vi "RT main.vi"() -> ()   [LabVIEW 2018]
uses:
  <vilib>/userdefined/High Color/nirio_resource_hc.ctl
  controls/Controller Data.ctl
  RT-FPGA Interface API/RT-FPGA Interface API.lvlib
panel:
  out "# pending remove":i32
  out "# elements in queue":i32
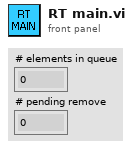
[diagram p1: front panel]
types:
  T1 = typedef "Controller Data.ctl" = cluster{"Closed Loop Enabled":bool, "Proportional valve 1":dbl, "Proportional valve 2":dbl, "Plant Control Variables":cluster{"Tank 1 Level":dbl, "Tank 2 Level":dbl, "Tank 3 Level":dbl, "Tank 4 Level":dbl, "Pump 1":dbl, "Pump 2":dbl}, "Setpoints":cluster{"Setpoint tank 1":dbl, "Setpoint tank 2":dbl}, "Controller":cluster{"A":dbl[][], "B":dbl[][], "C":dbl[][], "D":dbl[][]}}
  T2 = typedef "nirio_resource_hc.ctl" = tag
  T3 = typedef "RT-FPGA Interface API.lvlib/FPGA ref.ctl" = refnum<k20>
  T4 = cluster{"Proportional valve 1":dbl, "Proportional valve 2":dbl, "Pump 1":dbl, "Pump 2":dbl}
  T5 = cluster{"Setpoint Tank 1":dbl, "Setpoint Tank 2":dbl}
  T6 = cluster{"A":dbl[][], "B":dbl[][], "C":dbl[][], "D":dbl[][]}
  T7 = cluster{"Setpoint tank 1":dbl, "Setpoint tank 2":dbl}
  T8 = cluster{"Tank 1 Level":dbl, "Tank 2 Level":dbl, "Tank 3 Level":dbl, "Tank 4 Level":dbl, "Pump 1":dbl, "Pump 2":dbl}
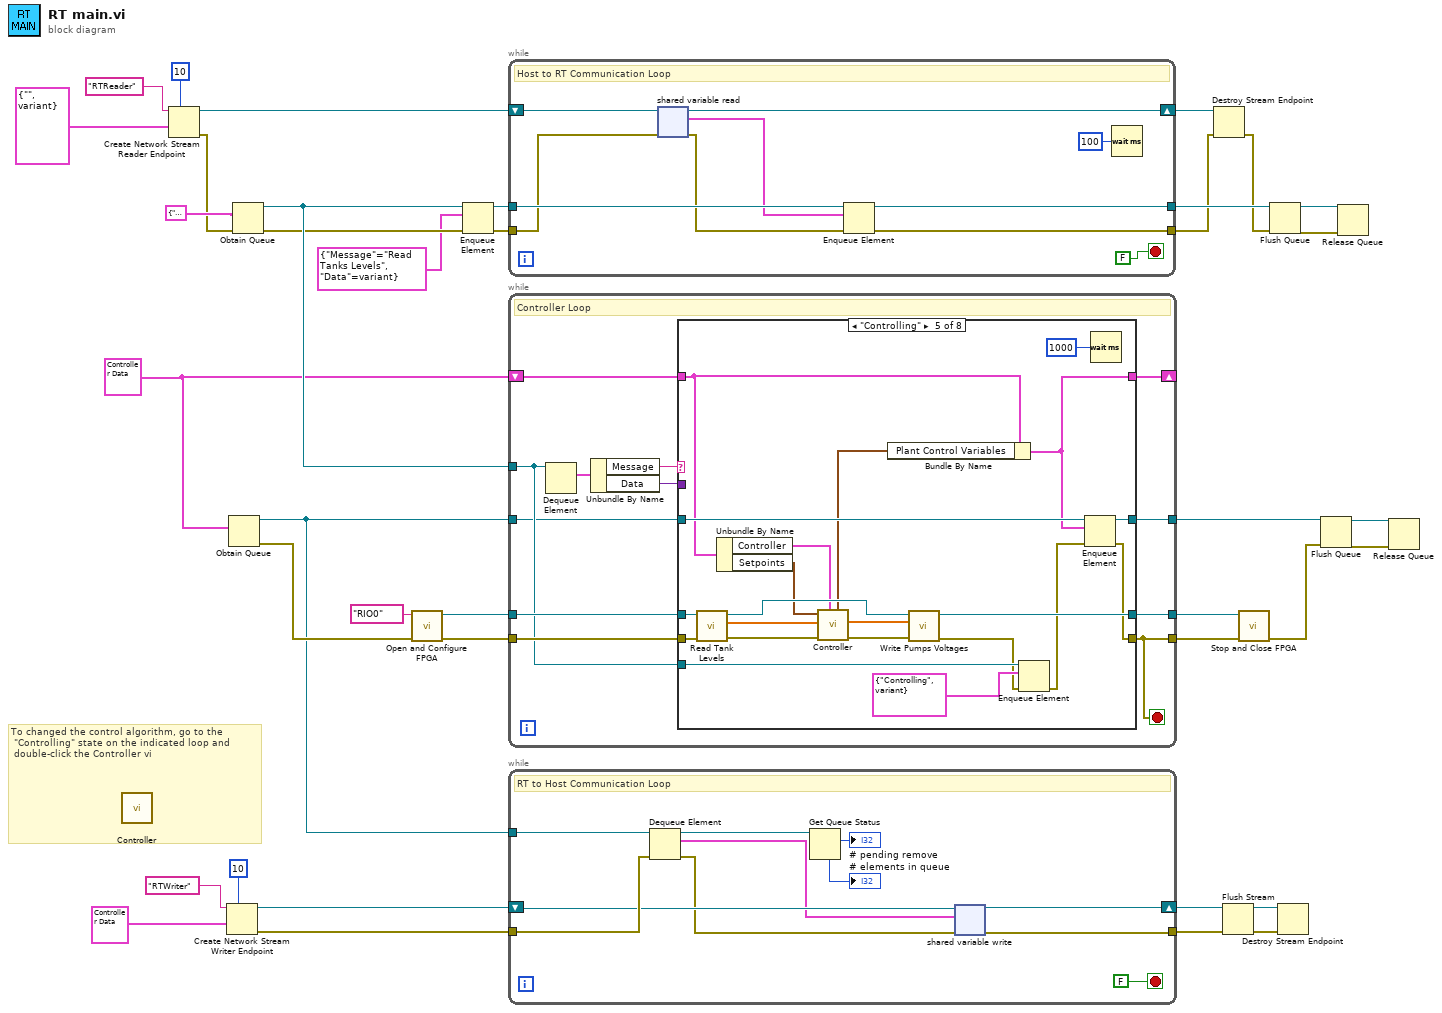
[diagram p0: block diagram]
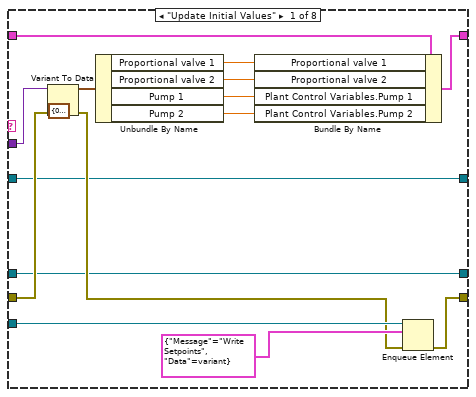
[diagram p2: hidden frame]
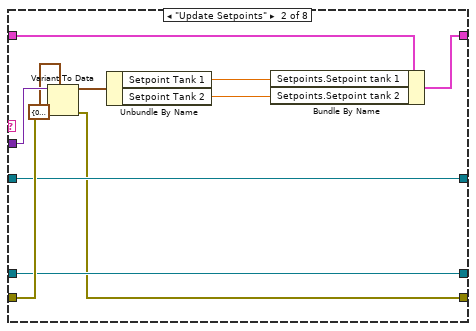
[diagram p3: hidden frame]
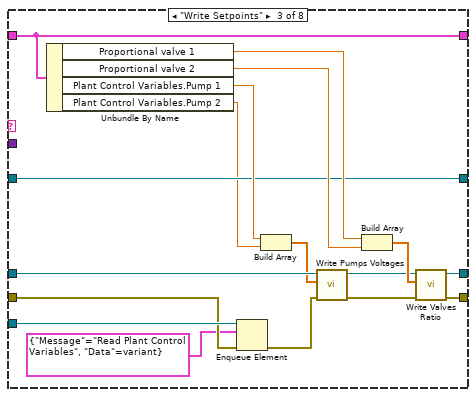
[diagram p4: hidden frame]
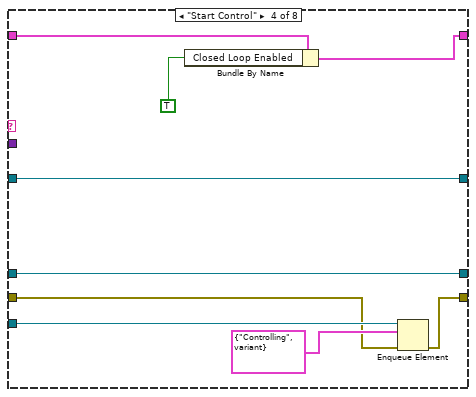
[diagram p5: hidden frame]
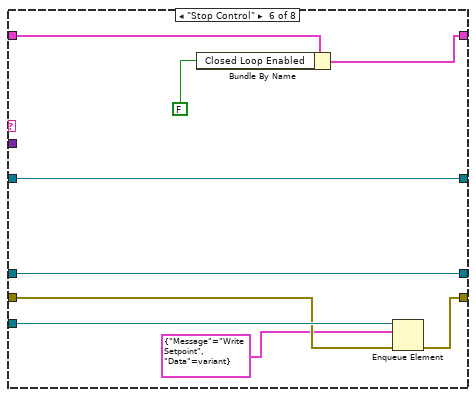
[diagram p6: hidden frame]
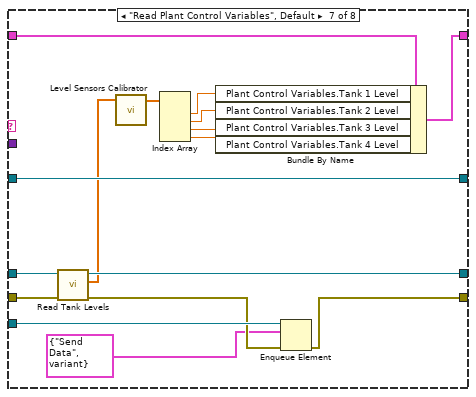
[diagram p7: hidden frame]
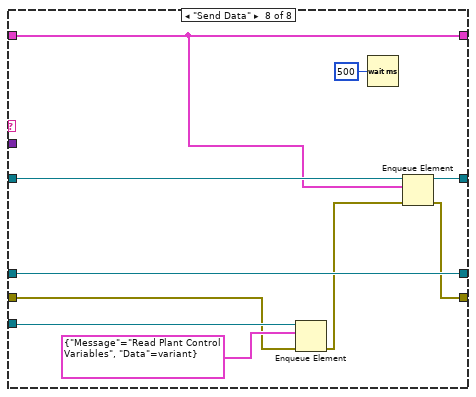
[diagram p8: hidden frame]
diagram:
  w2 = T1 {"Closed Loop Enabled"=FALSE, "Proportional valve 1"=0.0, "Proportional valve 2"=0.0, "Plant Control Variables"={"Tank 1 Level"=0.0, "Tank 2 Level"=0.0, "Tank 3 Level"=0.0, "Tank 4 Level"=0.0, "Pump 1"=0.0, "Pump 2"=0.0}, "Setpoints"={"Setpoint tank 1"=0.0, "Setpoint tank 2"=0.0}, "Controller"={"A"=[[-4.94989, 0.0218181, -352.966, 23.8192, -3.10685, -0.000952287], [-0.0218181, -4.904857, 23.4819, -343.472, 0.000977323, -3.58066], [0.0389045, 0.0, -31.6573, 0.0287797, 0.0245405, 0.0], [0.0, 0.0381972, 0.0287797, -31.6573, 0.0, 0.0280468], [0.0, 0.0325383, 0.0240248, -0.0293675, -0.0245405, 0.0], [0.031831, 0.0, -0.0282058, 0.0, 0.0, 0.0]], "B"=[[28.0692, -23.9099], [-23.3912, 28.5852], [31.6468, -0.0287797], [-0.0287797, 31.6468], [-0.0282058, -0.0293675], [0.0282058, -0.0240214]], "C"=[[4.94989, 0.0218181, 314.896, 0.0907351, 3.10685, 0.000952287], [10.0218181, 4.90457, -0.0906726, 314.884, -0.000977323, 3.58066]], "D"=[[0.0, 0.0], [0.0, 0.0]]}}
  # "To changed the control algorithm, go to the\n \"Controlling\" state on the indicated loop and\n double-click the Controller vi"
  n1 = call "Controller.vi"() -> ()  [unwired: 9 in, 3 out]
  n2 = Create Network Stream Reader Endpoint(7:10 ("writer buffer size"), 9:cluster{"Message":string, "Data":variant} {"Message"="", "Data"=variant} ("cluster"), 11:"RTReader" ("writer name")) -> (0:w5:errorcluster, 3:w30:refnum<k21>)  [unwired: 4 in]
  n3 = Create Network Stream Writer Endpoint(7:10 ("writer buffer size"), 9:T1 {"Closed Loop Enabled"=FALSE, "Proportional valve 1"=0.0, "Proportional valve 2"=0.0, "Plant Control Variables"={"Tank 1 Level"=0.0, "Tank 2 Level"=0.0, "Tank 3 Level"=0.0, "Tank 4 Level"=0.0, "Pump 1"=0.0, "Pump 2"=0.0}, "Setpoints"={"Setpoint tank 1"=0.0, "Setpoint tank 2"=0.0}, "Controller"={"A"=[[-4.94989, 0.0218181, -352.966, 23.8192, -3.10685, -0.000952287], [-0.0218181, -4.904857, 23.4819, -343.472, 0.000977323, -3.58066], [0.0389045, 0.0, -31.6573, 0.0287797, 0.0245405, 0.0], [0.0, 0.0381972, 0.0287797, -31.6573, 0.0, 0.0280468], [0.0, 0.0325383, 0.0240248, -0.0293675, -0.0245405, 0.0], [0.031831, 0.0, -0.0282058, 0.0, 0.0, 0.0]], "B"=[[28.0692, -23.9099], [-23.3912, 28.5852], [31.6468, -0.0287797], [-0.0287797, 31.6468], [-0.0282058, -0.0293675], [0.0282058, -0.0240214]], "C"=[[4.94989, 0.0218181, 314.896, 0.0907351, 3.10685, 0.000952287], [10.0218181, 4.90457, -0.0906726, 314.884, -0.000977323, 3.58066]], "D"=[[0.0, 0.0], [0.0, 0.0]]}}, 11:"RTWriter" ("writer name")) -> (0:w10:errorcluster, 3:w11:refnum<k21>)  [unwired: 4 in]
  n4 = Obtain Queue(element data type=w2) -> (queue out=w14:refnum<queue>, error out=w16:errorcluster)  [unwired: 4 in, 1 out]
  n5 = Obtain Queue(element data type=cluster{"Message":string, "Data":variant} {"Message"="", "Data"=variant} ("cluster"), error in (no error)=w5) -> (queue out=w22:refnum<queue>, error out=w21:errorcluster)  [unwired: 3 in, 1 out]
  n6 = call "Open and Configure FPGA.vi"("error in"=w16, "resource name"=T2 "RIO0") -> ("error out"=w37:errorcluster, "FPGA VI Reference Out"=w38:T3)  [unwired: 8 in]
  n7 = Enqueue Element(queue=w22, element=cluster{"Message":string, "Data":variant} {"Message"="Read Tanks Levels", "Data"=variant}, error in (no error)=w21) -> (queue out=w24:refnum<queue>, error out=w23:errorcluster)  [unwired: 1 in, 1 out]
  n8 = while {
    tunnel: w24 -> [w46]
    tunnel: [w45] -> w28
    tunnel: w23 -> [w42]
    tunnel: [w43] -> w4
    shift-right: [w47] -> w29
    shift-left: w30 -> [w48]
    stop <- FALSE stop-if-true
    # "Host to RT Communication Loop"
    n9 = shared-variable-read(w48, w42) -> (w47:refnum<k21>, w41:errorcluster, w44:cluster{"Message":string, "Data":variant})  [unwired: 1 in, 1 out]
    n10 = Enqueue Element(queue=w46, element=w44, error in (no error)=w41) -> (queue out=w45:refnum<queue>, error out=w43:errorcluster)  [unwired: 1 in, 1 out]
    n11 = Wait (ms)(milliseconds to wait=u32 100) -> ()  [unwired: 1 out]
  }
  n12 = while {
    tunnel: w38 -> [w60]
    tunnel: w37 -> [w59]
    tunnel: [w58] -> w36
    tunnel: [w49] -> w35
    tunnel: w22 -> [w52]
    shift-right: [w53] -> _
    shift-left: w2 -> [w54]
    tunnel: w14 -> [w51]
    tunnel: [w50] -> w17
    stop <- w49 stop-if-true
    # "Controller Loop"
    n13 = Dequeue Element(queue=w52) -> (element=w57:cluster{"Message":string, "Data":variant})  [unwired: 2 in, 3 out]
    n14 = Unbundle By Name(w57) -> ("Message"=w56:string, "Data"=w55:variant)
    n15 = case shown="\"Controlling\"" w56 {
      tunnel: w60 -> [w65 w83 w101 w111 w134 w141 w159 w169]
      tunnel: w59 -> [w72 w84 w90 w109 w133 w142 w158 w163]
      tunnel: [w65 w83 w103 w111 w132 w141 w157 w169] -> w58
      tunnel: [w68 w77 w102 w110 w119 w140 w147 w166] -> w49
      tunnel: w55 -> [w64 w82 _ _ _ _ _ _]
      tunnel: w54 -> [w73 w85 w100 w107 w121 w137 w149 w160]
      tunnel: [w74 w86 w100 w105 w116 w135 w148 w160] -> w53
      tunnel: w52 -> [w70 _ w91 w112 w131 w143 w156 w164]
      tunnel: w51 -> [w61 w81 w95 w108 w128 w138 w146 w168]
      tunnel: [w61 w81 w95 w108 w127 w138 w146 w167] -> w50
      frame "Update Initial Values" {
        n16 = Variant To Data(error in=w72, type=T4 {"Proportional valve 1"=0.0, "Proportional valve 2"=0.0, "Pump 1"=0.0, "Pump 2"=0.0} ("cluster"), Variant=w64) -> (data=w75:T4, error out=w69:errorcluster)
        n17 = Unbundle By Name(w75) -> ("Proportional valve 1"=w67:dbl, "Proportional valve 2"=w66:dbl, "Pump 1"=w63:dbl, "Pump 2"=w62:dbl)
        n18 = Bundle By Name(cluster=w73, "Proportional valve 1"=w67, "Proportional valve 2"=w66, "Plant Control Variables.Pump 1"=w63, "Plant Control Variables.Pump 2"=w62) -> (w74:T1)
        n19 = Enqueue Element(queue=w70, element=cluster{"Message":string, "Data":variant} {"Message"="Write Setpoints", "Data"=variant}, error in (no error)=w69) -> (error out=w68:errorcluster)  [unwired: 1 in, 2 out]
      }
      frame "Update Setpoints" {
        n20 = Variant To Data(error in=w84, type=T5 {"Setpoint Tank 1"=0.0, "Setpoint Tank 2"=0.0} ("cluster"), Variant=w82) -> (data=w87:T5, error out=w77:errorcluster)
        n21 = Unbundle By Name(w87) -> ("Setpoint Tank 1"=w79:dbl, "Setpoint Tank 2"=w78:dbl)
        n22 = Bundle By Name(cluster=w85, "Setpoints.Setpoint tank 1"=w79, "Setpoints.Setpoint tank 2"=w78) -> (w86:T1)
      }
      frame "Write Setpoints" {
        n23 = Unbundle By Name(w100) -> ("Proportional valve 1"=w98:dbl, "Proportional valve 2"=w97:dbl, "Plant Control Variables.Pump 1"=w99:dbl, "Plant Control Variables.Pump 2"=w94:dbl)
        n24 = Enqueue Element(queue=w91, element=cluster{"Message":string, "Data":variant} {"Message"="Read Plant Control Variables", "Data"=variant}, error in (no error)=w90) -> (error out=w92:errorcluster)  [unwired: 1 in, 2 out]
        n25 = Build Array(w99, w94) -> (w93:dbl[])
        n26 = call "Write Pumps Voltages.vi"("error in (no error)"=w92, "Pumps Voltages"=w93, "FPGA VI Reference In"=w101) -> ("error out"=w104:errorcluster, "FPGA VI Reference Out"=w88:T3)  [unwired: 7 in]
        n27 = Build Array(w98, w97) -> (w96:dbl[])
        n28 = call "Write Valves Ratio.vi"("error in (no error)"=w104, "Valves ratios"=w96, "FPGA VI Reference In"=w88) -> ("error out"=w102:errorcluster, "FPGA VI Reference Out"=w103:T3)  [unwired: 7 in]
      }
      frame "Start Control" {
        n29 = Bundle By Name(cluster=w107, "Closed Loop Enabled"=TRUE) -> (w105:T1)
        n30 = Enqueue Element(queue=w112, element=cluster{"Message":string, "Data":variant} {"Message"="Controlling", "Data"=variant}, error in (no error)=w109) -> (error out=w110:errorcluster)  [unwired: 1 in, 2 out]
      }
      frame "Controlling" {
        n31 = call "Read Tank Levels.vi"("error in (no error)"=w133, "FPGA VI Reference In"=w134) -> ("error out"=w124:errorcluster, "Tanks levels"=w125:dbl[], "FPGA VI Reference Out"=w126:T3)  [unwired: 7 in]
        n32 = Unbundle By Name(w121) -> ("Controller"=w114:T6, "Setpoints"=w120:T7)
        n33 = call "Controller.vi"("State-Space"=w114, "error in (no error)"=w124, "Tanks levels"=w125, "Setpoints"=w120) -> ("error out"=w123:errorcluster, "Pumps Voltages"=w122:dbl[], "Plant Control Variables"=w115:T8)  [unwired: 5 in]
        n34 = Bundle By Name(cluster=w121, "Plant Control Variables"=w115) -> (w116:T1)
        n35 = call "Write Pumps Voltages.vi"("error in (no error)"=w123, "Pumps Voltages"=w122, "FPGA VI Reference In"=w126) -> ("error out"=w117:errorcluster, "FPGA VI Reference Out"=w132:T3)  [unwired: 7 in]
        n36 = Enqueue Element(queue=w131, element=cluster{"Message":string, "Data":variant} {"Message"="Controlling", "Data"=variant}, error in (no error)=w117) -> (error out=w118:errorcluster)  [unwired: 1 in, 2 out]
        n37 = Enqueue Element(queue=w128, element=w116, error in (no error)=w118) -> (queue out=w127:refnum<queue>, error out=w119:errorcluster)  [unwired: 1 in, 1 out]
        n38 = Wait (ms)(milliseconds to wait=u32 1000) -> ()  [unwired: 1 out]
      }
      frame "Stop Control" {
        n39 = Bundle By Name(cluster=w137, "Closed Loop Enabled"=FALSE) -> (w135:T1)
        n40 = Enqueue Element(queue=w143, element=cluster{"Message":string, "Data":variant} {"Message"="Write Setpoint", "Data"=variant}, error in (no error)=w142) -> (error out=w140:errorcluster)  [unwired: 1 in, 2 out]
      }
      frame "Read Plant Control Variables", Default {
        n41 = call "Read Tank Levels.vi"("error in (no error)"=w158, "FPGA VI Reference In"=w159) -> ("error out"=w155:errorcluster, "Tanks levels"=w145:dbl[], "FPGA VI Reference Out"=w157:T3)  [unwired: 7 in]
        n42 = call "Level Sensors Calibrator.vi"("Data in"=w145) -> ("Data out"=w144:dbl[])  [unwired: 4 in]
        n43 = Index Array(array=w144) -> (element #1=w152:dbl, element #2=w151:dbl, element #3=w150:dbl, element #4=w153:dbl)  [unwired: 4 in]
        n44 = Bundle By Name(cluster=w149, "Plant Control Variables.Tank 1 Level"=w152, "Plant Control Variables.Tank 2 Level"=w151, "Plant Control Variables.Tank 3 Level"=w150, "Plant Control Variables.Tank 4 Level"=w153) -> (w148:T1)
        n45 = Enqueue Element(queue=w156, element=cluster{"Message":string, "Data":variant} {"Message"="Send Data", "Data"=variant}, error in (no error)=w155) -> (error out=w147:errorcluster)  [unwired: 1 in, 2 out]
      }
      frame "Send Data" {
        n46 = Enqueue Element(queue=w164, element=cluster{"Message":string, "Data":variant} {"Message"="Read Plant Control Variables", "Data"=variant}, error in (no error)=w163) -> (error out=w162:errorcluster)  [unwired: 1 in, 2 out]
        n47 = Wait (ms)(milliseconds to wait=u32 500) -> ()  [unwired: 1 out]
        n48 = Enqueue Element(queue=w168, element=w160, error in (no error)=w162) -> (queue out=w167:refnum<queue>, error out=w166:errorcluster)  [unwired: 1 in, 1 out]
      }
    }
  }
  n49 = while {
    tunnel: w14 -> [w174]
    tunnel: w10 -> [w180]
    tunnel: [w176] -> w6
    shift-right: [w177] -> w7
    shift-left: w11 -> [w179]
    stop <- FALSE stop-if-true
    # "RT to Host Communication Loop"
    n50 = Dequeue Element(queue=w174, error in (no error)=w180) -> (queue out=w172:refnum<queue>, element=w170:T1, error out=w178:errorcluster)  [unwired: 1 in, 1 out]
    n51 = Get Queue Status(queue=w172) -> (# pending remove=→"# pending remove":i32, # elements in queue=→"# elements in queue":i32)  [unwired: 2 in, 6 out]
    n52 = shared-variable-write(w179, w178, w170) -> (w177:refnum<k21>, w176:errorcluster)  [unwired: 1 in, 1 out]
  }
  n53 = Destroy Stream Endpoint(8:w4, 11:w29) -> (0:w3:errorcluster)
  n54 = Flush Stream(8:w6, 11:w7) -> (0:w8:errorcluster, 3:w9:refnum<k21>)  [unwired: 2 in, 1 out]
  n55 = call "Stop and Close FPGA.vi"("error in (no error)"=w35, "FPGA VI Reference In"=w36) -> ("error out"=w15:errorcluster)  [unwired: 9 in]
  n56 = Flush Queue(queue=w28, error in (no error)=w3) -> (queue out=w27:refnum<queue>, error out=w26:errorcluster)  [unwired: 1 out]
  n57 = Destroy Stream Endpoint(8:w8, 11:w9) -> ()  [unwired: 1 out]
  n58 = Flush Queue(queue=w17, error in (no error)=w15) -> (queue out=w19:refnum<queue>, error out=w18:errorcluster)  [unwired: 1 out]
  n59 = Release Queue(queue=w27, error in (no error)=w26) -> ()  [unwired: 1 in, 3 out]
  n60 = Release Queue(queue=w19, error in (no error)=w18) -> ()  [unwired: 1 in, 3 out]
